vi "TalkTracker_Single.vi"(0 "PORT NAME":string="Inlet_Heaters", 1 "Set":enum16{"Set", "Read"}(ring), 3 "Value to set":dbl, 9 "LOCATION":i32=15, 11 "NO. LOCATIONS":i32=1, 12 "Analogue":enum16{"Logic", "Analogue"}(ring)) -> ()   [LabVIEW 2010]
panel:
  out "Module Address":i32
  out "Comment out":string
  out "Response":string=" ON\r\n"
  in  "Heater Number":i32=1 min=1 max=15
  in  "Module Addresses":i32[](array[numeric])=[101, 102, 103, 104, 105, 106, 107, 108, 109, 110, 111, 112, 113, 114, 115]
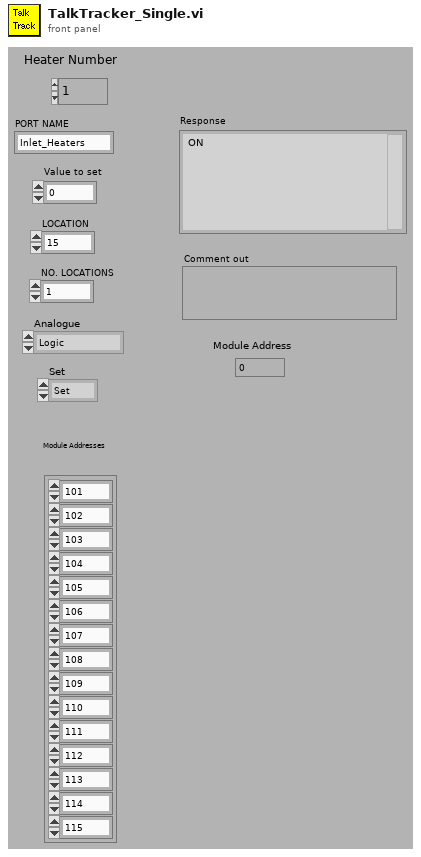
[diagram p1: front panel]
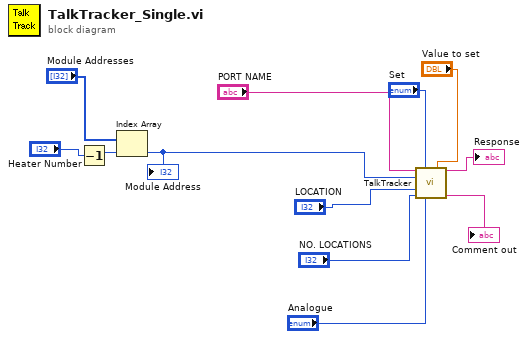
[diagram p0: block diagram]
diagram:
  n1 = Decrement(x="Heater Number") -> (x-1=w4:i32)
  n2 = Index Array(array="Module Addresses", index=w4) -> (element=w1:i32)
  "Module Address" <- w1
  n3 = call "TalkTracker.vi"("PORT NAME"="PORT NAME", "Set"="Set", "Value to set"="Value to set", "MODULE ADDRESS"=w1, "LOCATION"="LOCATION", "NO. LOCATIONS"="NO. LOCATIONS", "Analogue"="Analogue") -> ("Response"=→"Response":string, "Comment out"=→"Comment out":string)  [unwired: 6 in, 1 out]
